vi "Process.vi"(8 "error in":errorcluster, 11 "Plugin in":refnum<class "RPM Plugin.lvclass">) -> (0 "error out":errorcluster, 3 "Plugin out":refnum<class "RPM Plugin.lvclass">)   [LabVIEW 2020, in "RPM Plugin.lvlib" / "RPM Plugin.lvclass"]
uses:
  RPM Plugin.lvclass
  C:/Program Files/National Instruments/LabVIEW 2020/vi.lib/FlexLogger/SDK/PluginSDK.lvlibp/PEFClasses/SDK/Plugin/Plugin.lvclass
  RPM Plugin.lvclass/RPM Plugin.ctl
  <vilib>/DAQmx/read.llb/DAQmx Read (Counter DBL 1Chan 1Samp).vi
  <vilib>/DAQmx/miscellaneous.llb/DAQmx Fill In Error Info.vi
  <vilib>/FlexLogger/SDK/PluginSDK.lvlibp/PEFClasses/SDK/Plugin/DataHelpers/Write 1D DBL (NChan 1Sample).vi
  <vilib>/FlexLogger/SDK/PluginSDK.lvlibp/PEFClasses/SDK/Plugin/Plugin.lvclass
  C:/Program Files/National Instruments/LabVIEW 2020/vi.lib/FlexLogger/SDK/PluginSDK.lvlibp/PEFClasses/SDK/Processing Element/Processing Element.lvclass
  D:/AE/Transportation/Schwing Stetter/RPM Plugin/RPM Plugin/RPM Plugin.lvclass
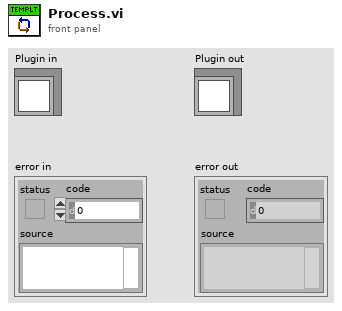
[diagram p1: front panel]
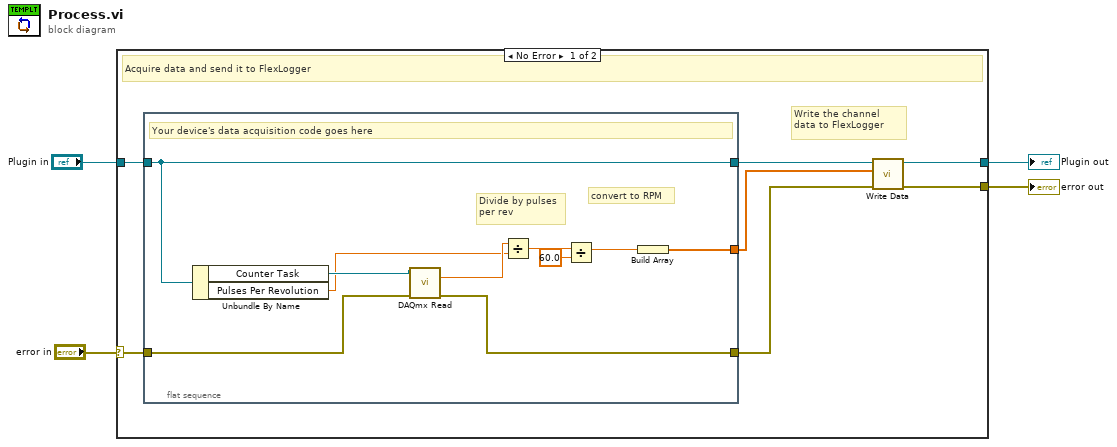
[diagram p0: block diagram]
diagram:
  n1 = case shown="No Error" "error in" {
    selector: "error in" -> [w10 w22]
    tunnel: [w6 w23] -> w4
    tunnel: "Plugin in" -> [w11 w23]
    tunnel: [w7 w22] -> w1
    frame No Error {
      # "Write the channel data to FlexLogger"
      # "Acquire data and send it to FlexLogger"
      n2 = flat-sequence {
        tunnel: [w12] -> w5
        tunnel: w11 -> [w21]
        tunnel: [w21] -> w9
        tunnel: w10 -> [w19]
        tunnel: [w18] -> w8
        frame #0 {
          # "Divide by pulses\nper rev"
          # "convert to RPM"
          # "Your device's data acquisition code goes here"
          n3 = Unbundle By Name(w21) -> ("Counter Task"=w20:refnum<k21>, "Pulses Per Revolution"=w16:dbl)
          n4 = call-poly <vilib>:"DAQmx Read.vi"("task/channels in"=w20, "error in"=w19) -> ("data"=w17:dbl, "error out"=w18:errorcluster)  [unwired: 11 in, 1 out]
          n5 = Divide(x=w17, y=w16) -> (x/y=w15:dbl)
          n6 = Divide(x=w15, y=60.0) -> (x/y=w13:dbl)
          n7 = Build Array(w13) -> (w12:dbl[])
        }
      }
      n8 = call-poly <vilib>:"Write Data.vi"("error in (no error)"=w8, "Data"=w5, "Plugin in"=w9) -> ("error out"=w7:errorcluster, "Plugin out"=w6:refnum<class "RPM Plugin.lvclass">)  [unwired: 7 in]
    }
    frame Error {
    }
  }
  "error out" <- w1
  "Plugin out" <- w4
